vi "MQTT HASS Subscriber.vi"() -> ()   [LabVIEW 2021]
uses:
  <vilib>/LabVIEW Open Source Project/MQTT Control Packets/Control Packets/CONNECT/ConnectFlags -- cluster.ctl
  <vilib>/LabVIEW Open Source Project/MQTT Client/Client class/Client.lvclass/Client.ctl
  <vilib>/LabVIEW Open Source Project/MQTT Client/Client class/Client.lvclass
  C:/Program Files (x86)/National Instruments/LabVIEW 2021/vi.lib/LabVIEW Open Source Project/MQTT Connection/MQTT_Base/Base Class/MQTT_Base.lvclass
  <vilib>/LabVIEW Open Source Project/Connection/Connection.TCP/Connection.TCP.lvclass
  C:/Program Files (x86)/National Instruments/LabVIEW 2021/vi.lib/LabVIEW Open Source Project/Connection/Connection/Connection.lvclass
  <vilib>/LabVIEW Open Source Project/MQTT Control Packets/Control Packets/PUBLISH/PUBLISH.lvclass
  <vilib>/LabVIEW Open Source Project/MQTT Connection/MQTT_Base/Base Class/MQTT_Base.lvclass
  <vilib>/LabVIEW Open Source Project/MQTT Control Packets/Control Packets/CONNECT/CONNECT.lvclass
  <vilib>/LabVIEW Open Source Project/MQTT Control Packets/Control Packets/ControlPacket/ControlPacket.lvclass
  <vilib>/JDP Science/JDP Science Common Utilities/JDP Utility.lvlib
  <vilib>/JDP Science/JSONtext/JSONtext.lvlib
panel:
  out "Received Topic":string="homeassistant/#"
  out "Voltage Chart":dbl(graph)
  out "Current Chart":dbl(graph)
  out "State String":string
  in  "State topic":string="lab/psu/state"
  out "Config String":string
  out "Connected?":bool
  in  "Config Topic":string="homeassistant/#"
  in  "remote port (1883)":u16=1883
  in  "address (localhost)":string="localhost"
  in  "STOP":bool
  # "(Simulation)"
  # "HASS Subscriber"
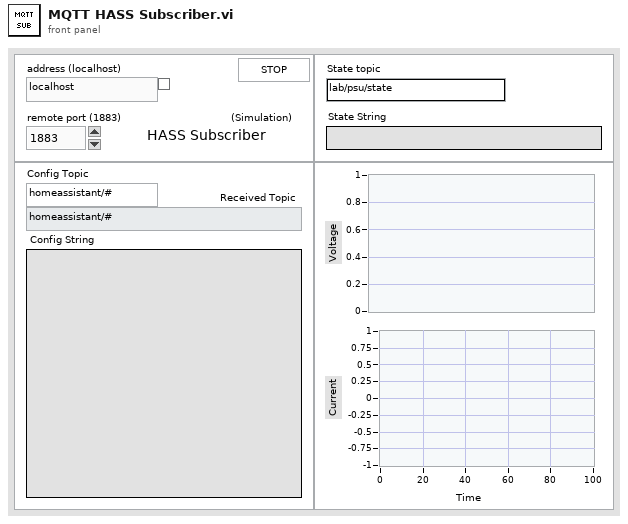
[diagram p1: front panel]
types:
  T1 = enum32{"Invalid", "Standard", "Closed", "Hidden", "Minimized", "Maximized"}
  T2 = enum32{"invalid app kind", "Development System", "Run Time System", "Student Edition", "Embedded LabVIEW", "Evaluation", "Custom"}
  T3 = cluster{"Will Topic":string, "Will Message":string, "Username":string, "Password":string}
  T4 = typedef "MQTT_Control_Packets.lvlib/CONNECT.lvclass/ConnectFlags -- cluster.ctl" = cluster{"Reserved":bool, "Clean Session":bool, "Will Flag":bool, "Will QoS 1":bool, "Will QoS 2":bool, "Will Retain":bool, "Password Flag":bool, "User Name Flag":bool}
  T5 = cluster{"Core":cluster{"Current VI Reference":refnum<vi>, "Close Panel on Exit?":bool}, "Connected?":bool}
  T6 = cluster{"Current VI Reference":refnum<vi>, "Close Panel on Exit?":bool}
  T7 = typedef "MQTT Client.lvlib/Client.lvclass/Public Events -- cluster.ctl" = cluster{"Connection Status":refnum<user-event>, "Connected":refnum<user-event>, "Application Message":refnum<user-event>}
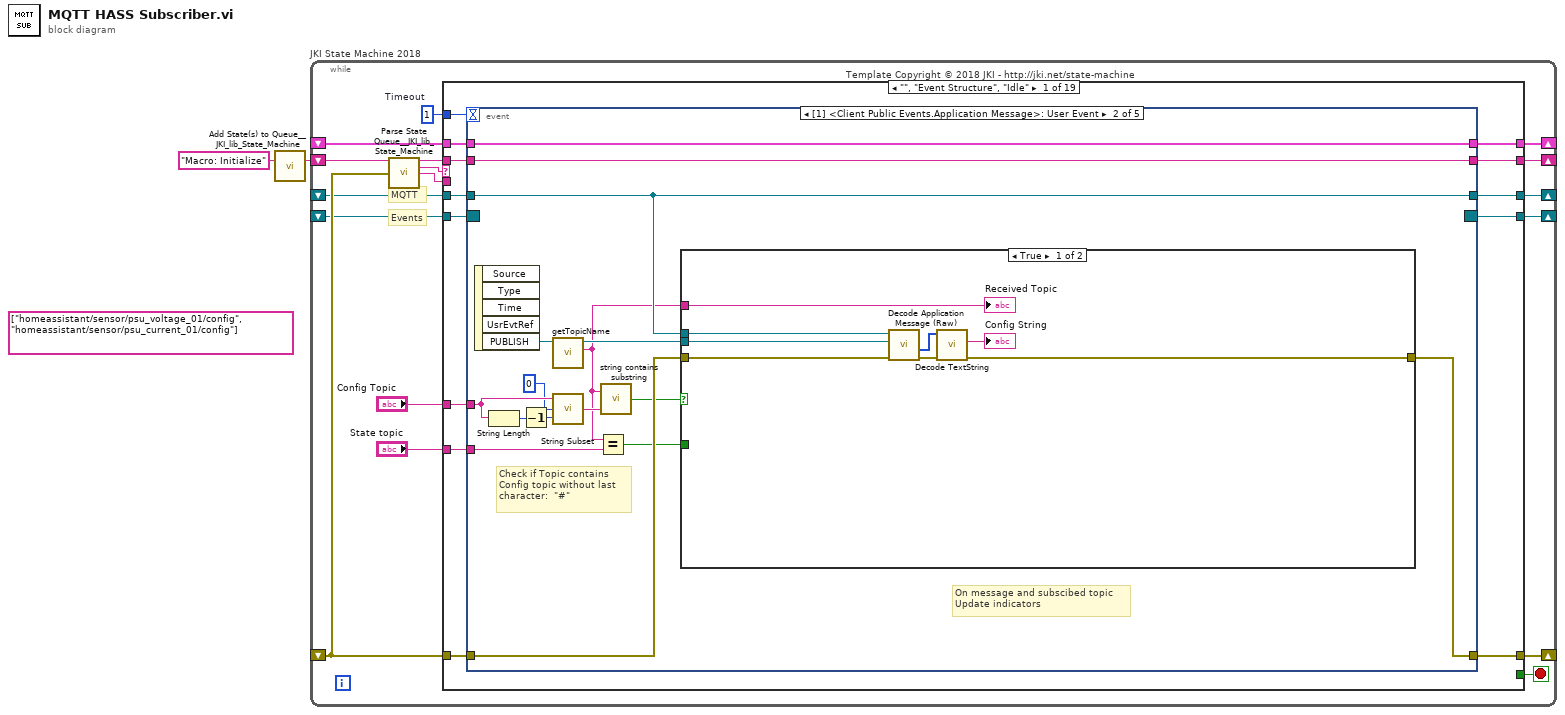
[diagram p0: block diagram]
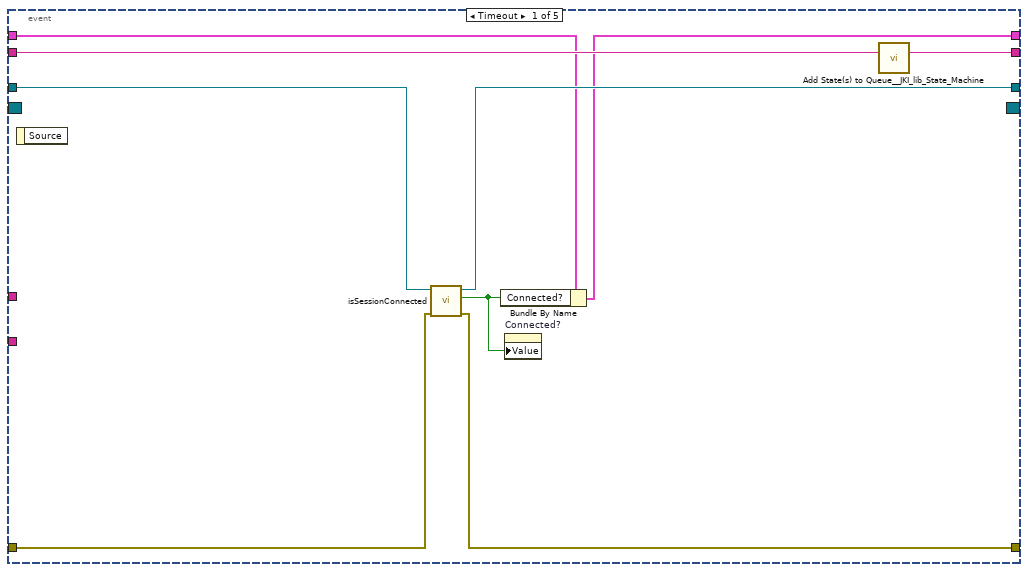
[diagram p2: hidden frame]
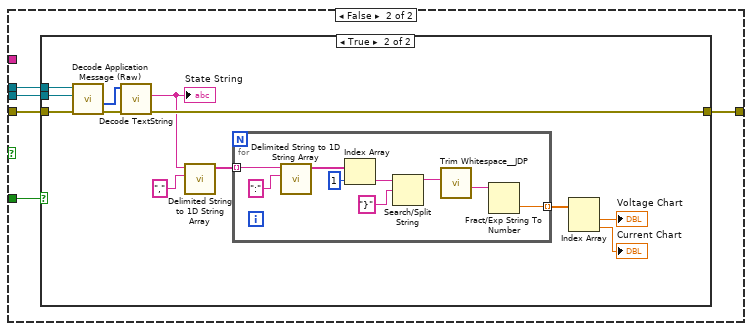
[diagram p3: hidden frame]
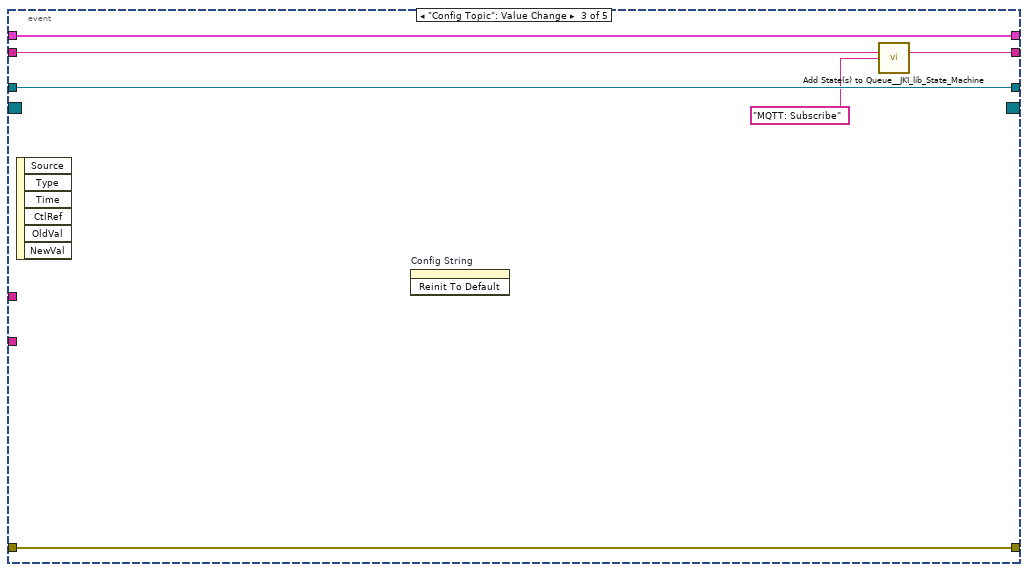
[diagram p5: hidden frame]
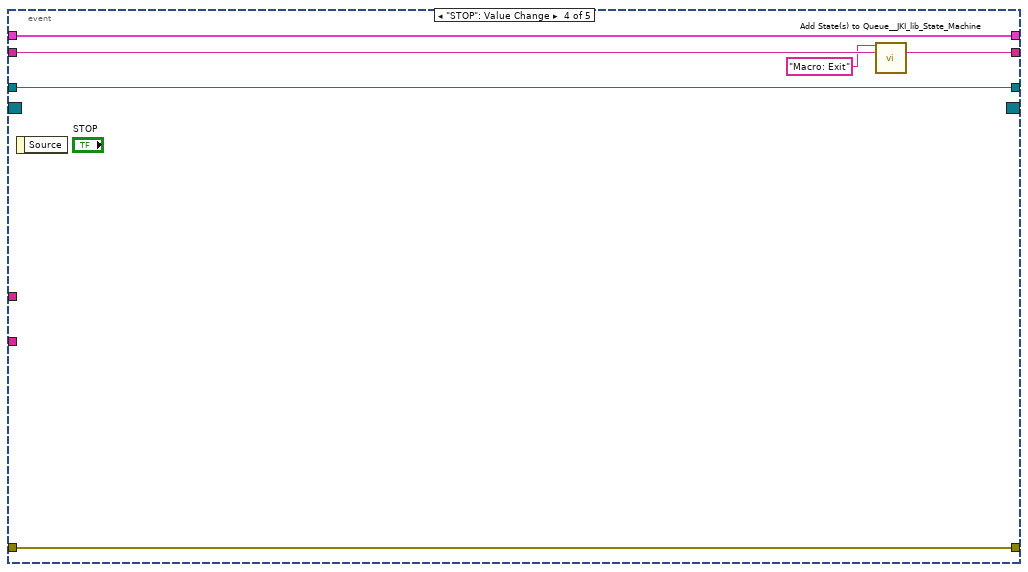
[diagram p6: hidden frame]
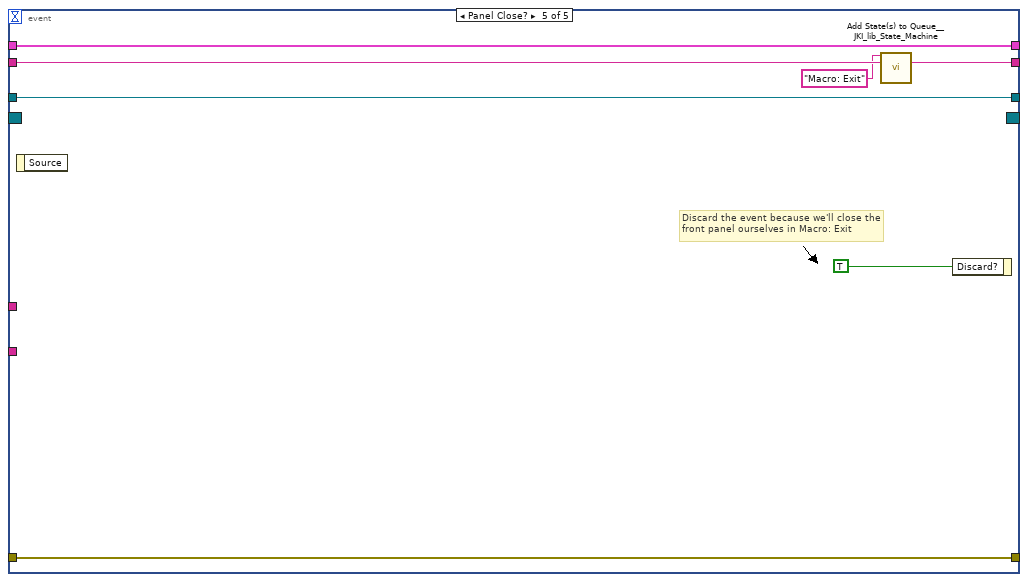
[diagram p7: hidden frame]
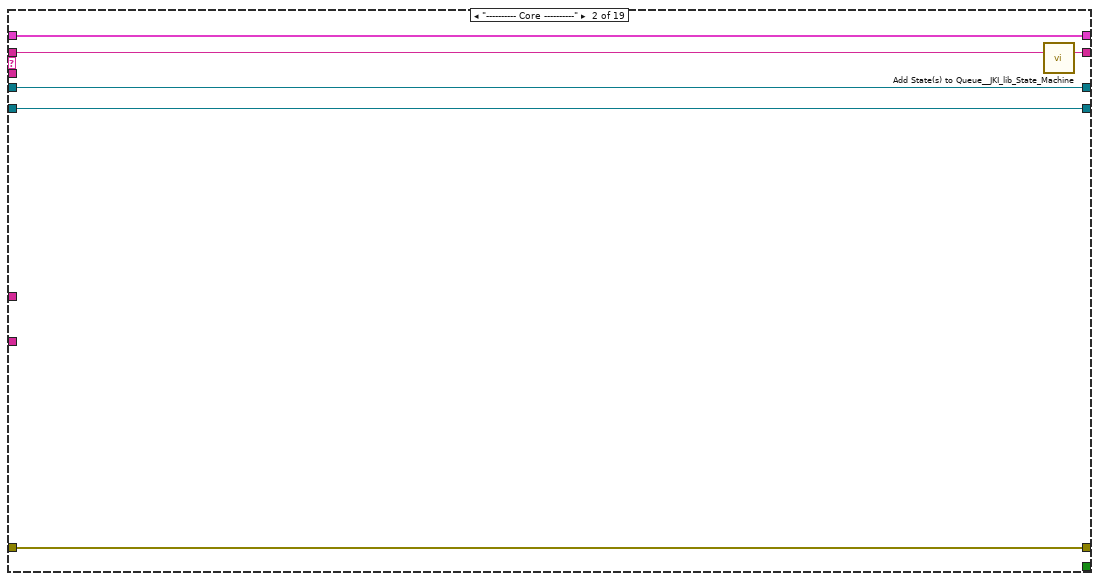
[diagram p8: hidden frame]
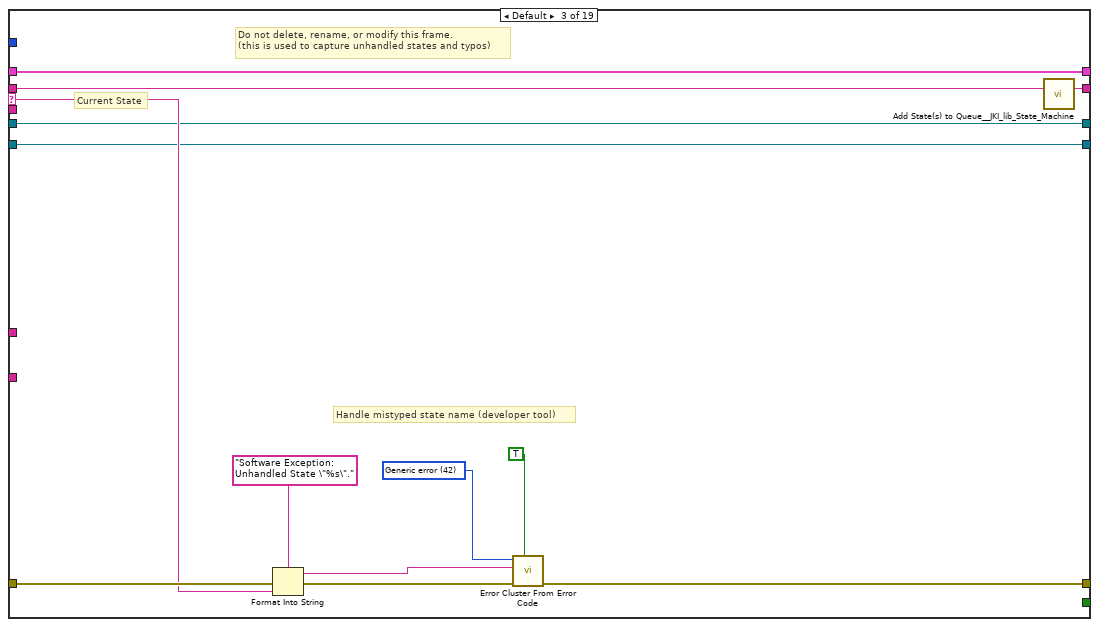
[diagram p9: hidden frame]
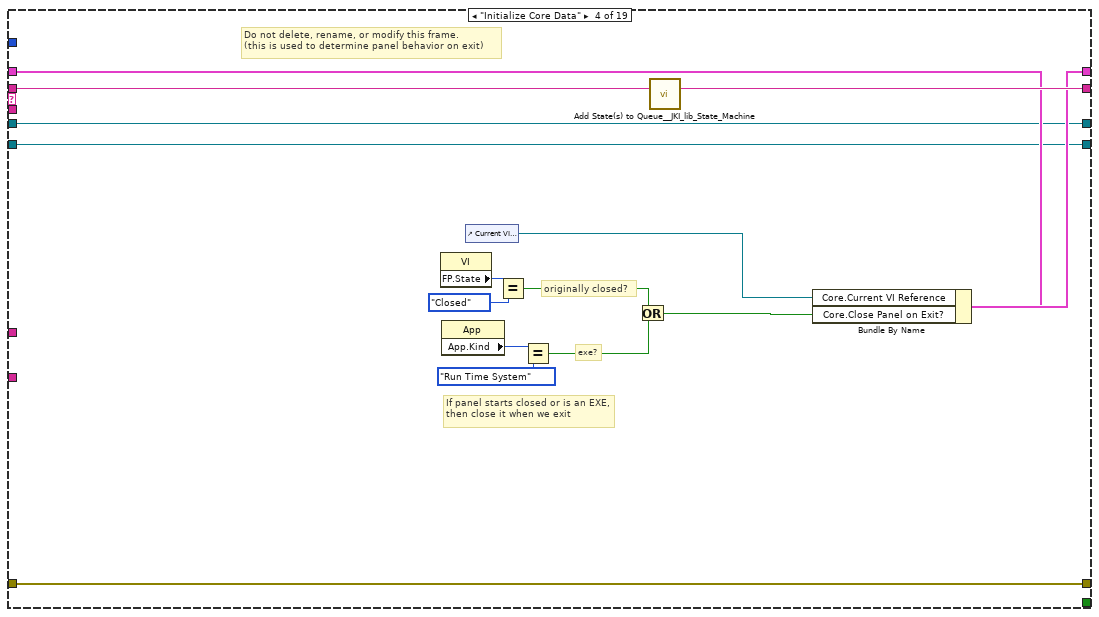
[diagram p10: hidden frame]
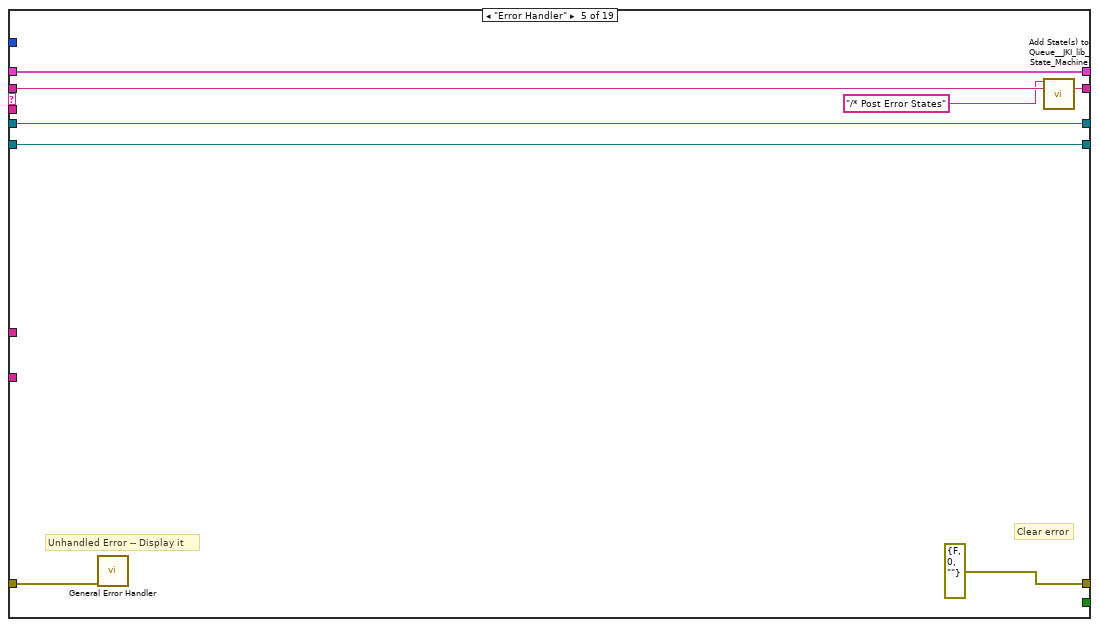
[diagram p11: hidden frame]
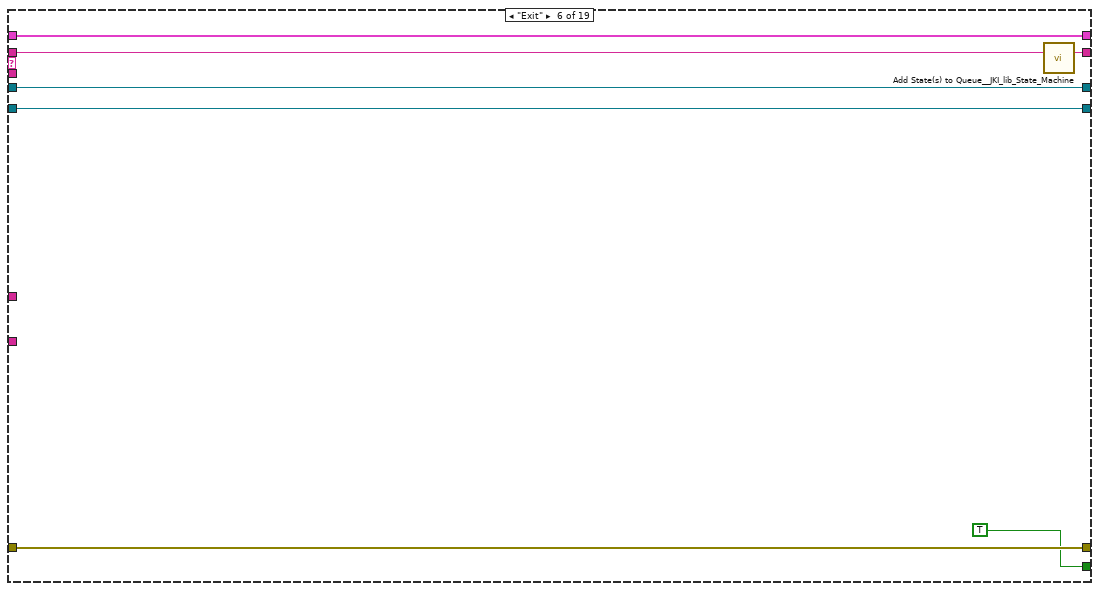
[diagram p12: hidden frame]
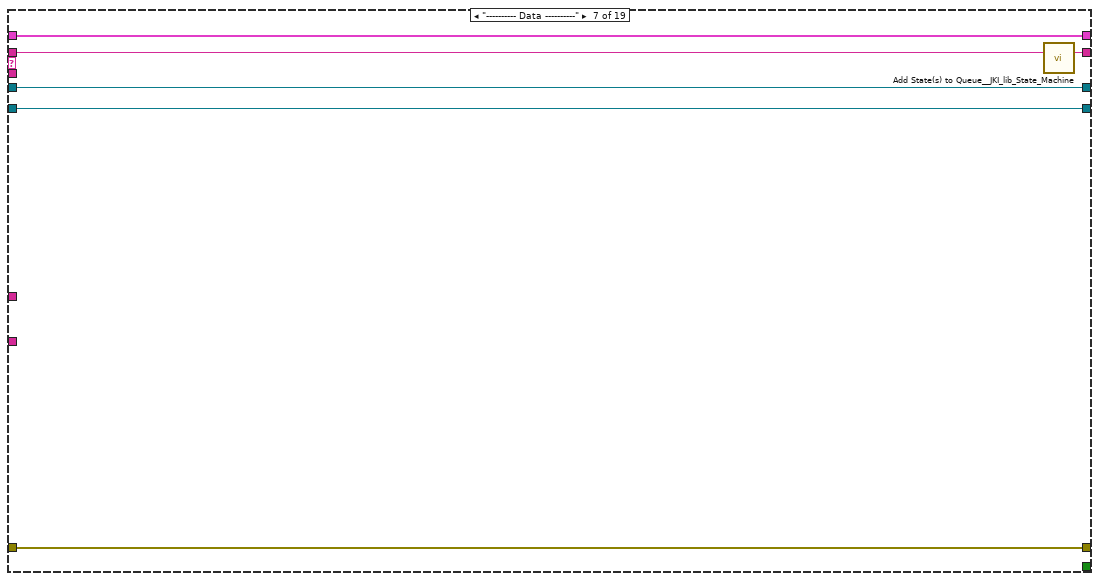
[diagram p13: hidden frame]
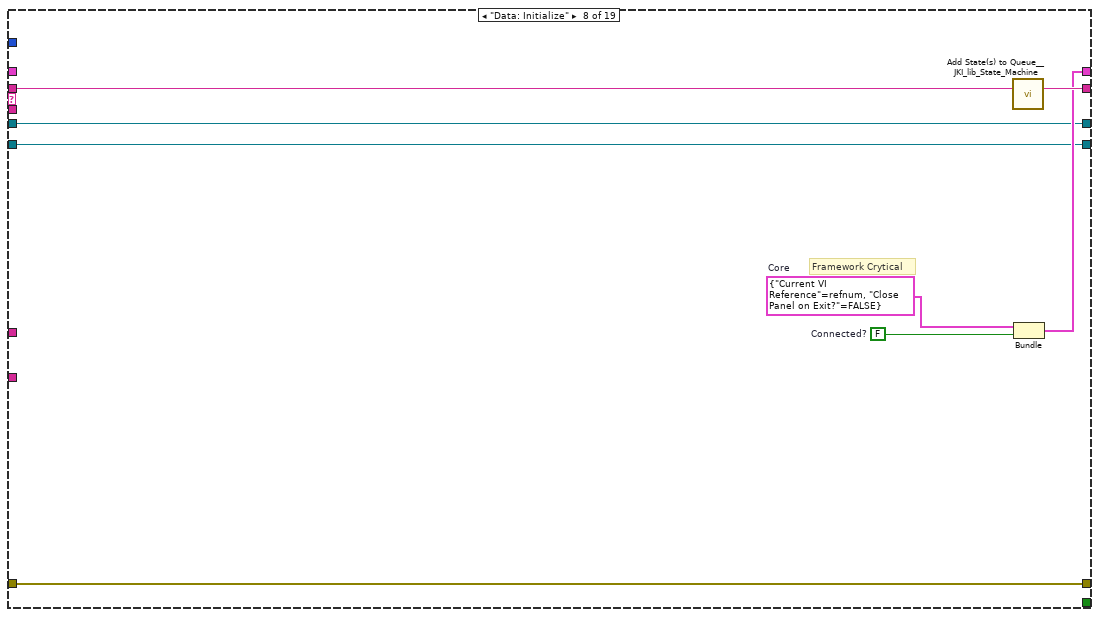
[diagram p14: hidden frame]
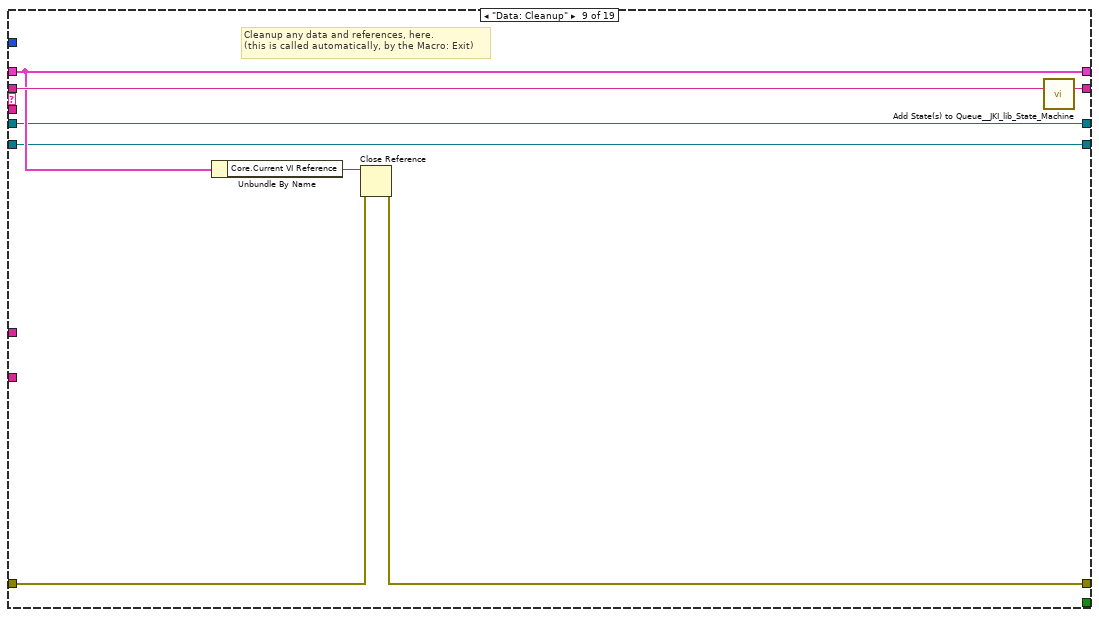
[diagram p15: hidden frame]
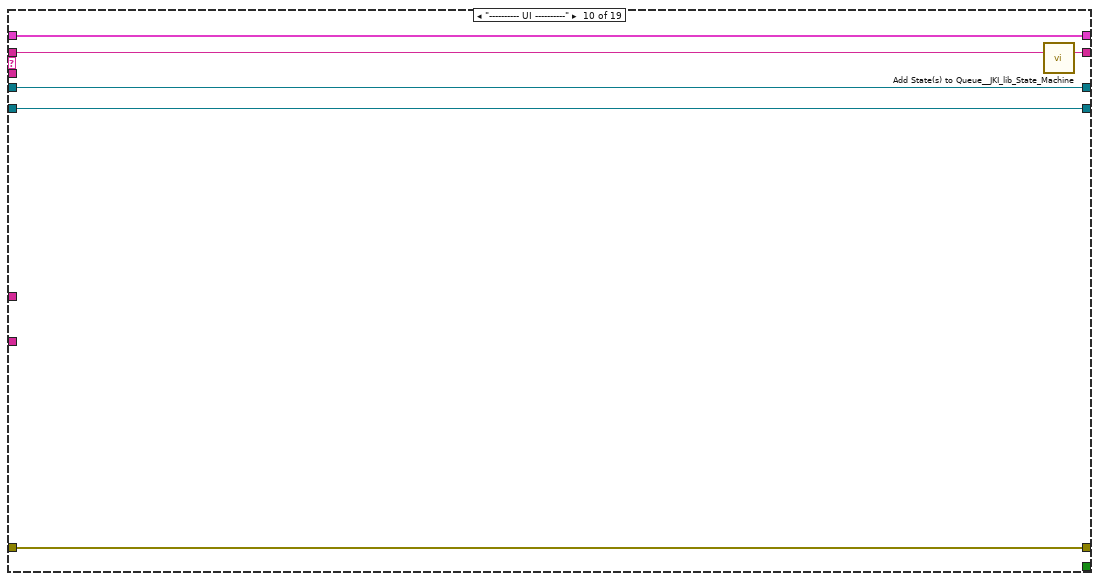
[diagram p16: hidden frame]
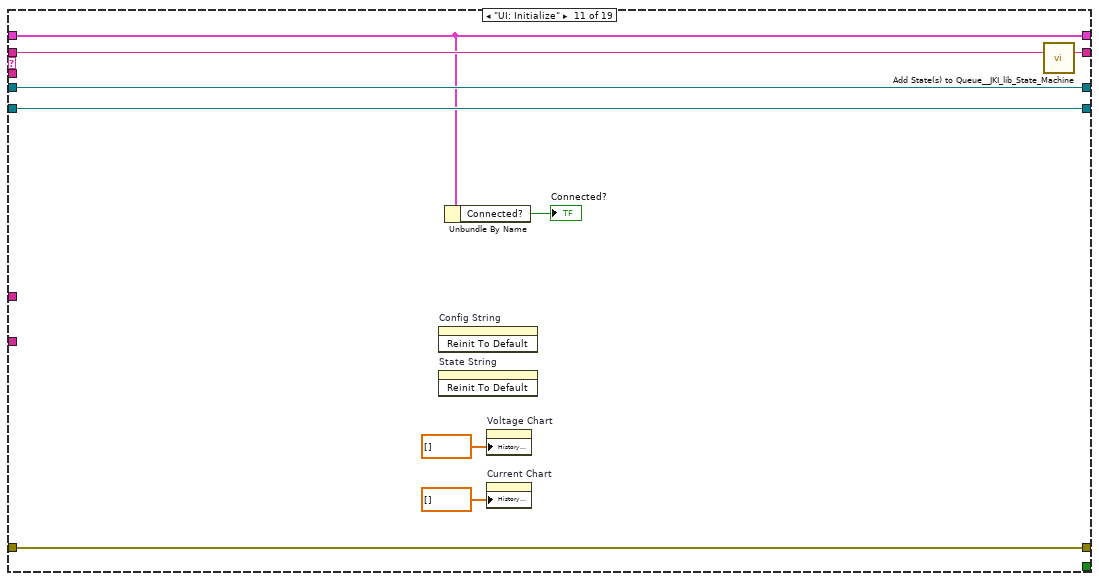
[diagram p17: hidden frame]
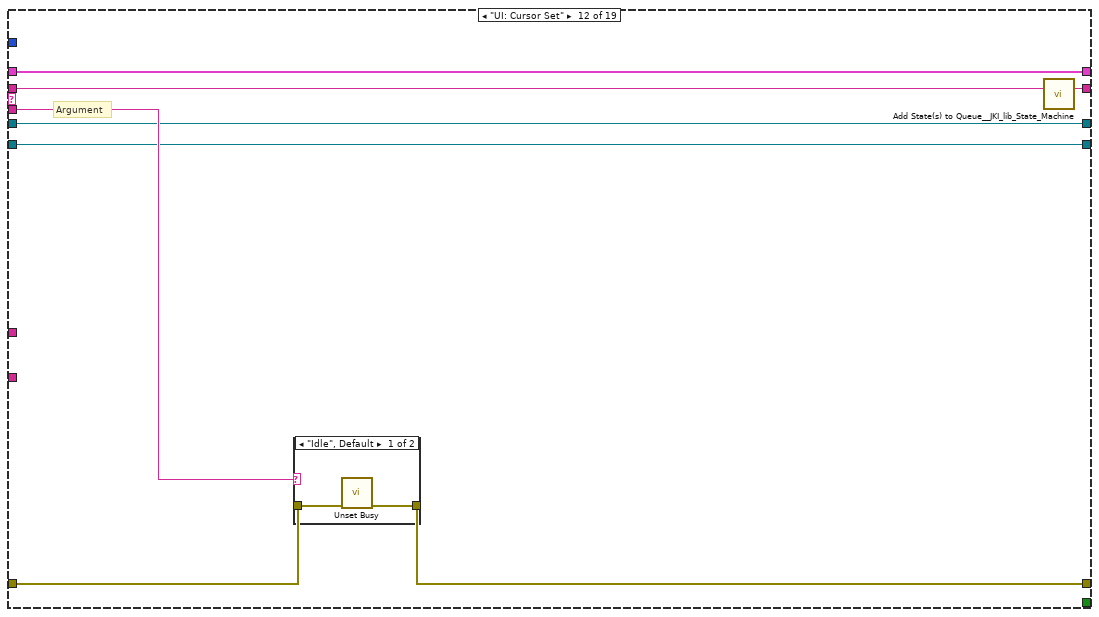
[diagram p18: hidden frame]
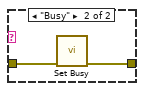
[diagram p19: hidden frame]
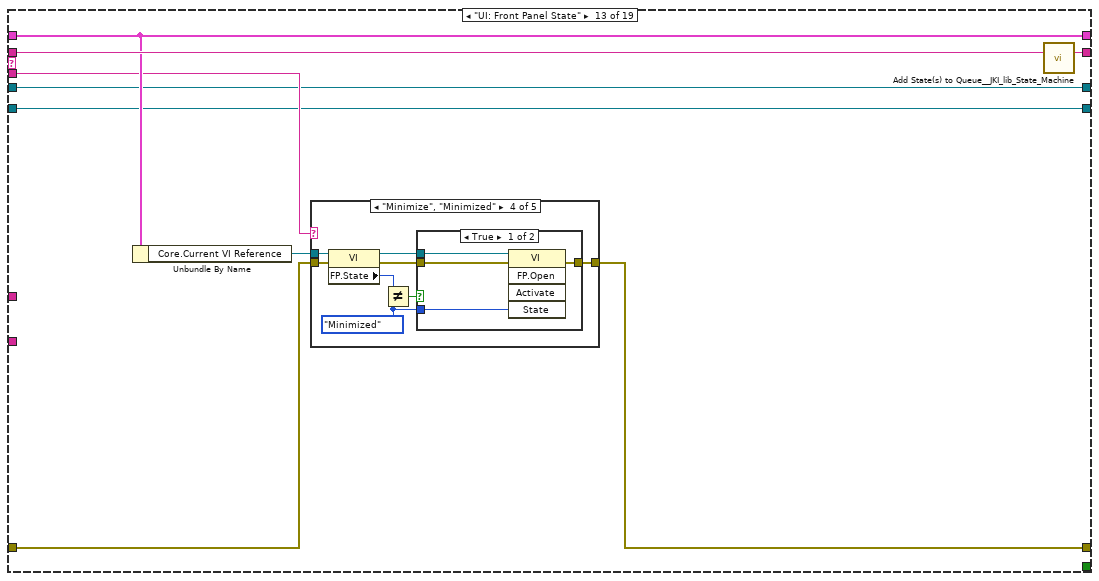
[diagram p20: hidden frame]
diagram:
  (unwired) string[] ["homeassistant/sensor/psu_voltage_01/config", "homeassistant/sensor/psu_current_01/config"]
  n1 = call <vilib>:"Add State(s) to Queue__JKI_lib_State_Machine.vi"("State(s) in (\"\")"="Macro: Initialize") -> ("States Out"=w2:string)  [unwired: 14 in]
  n2 = while "JKI State Machine 2018" {
    shift-right: [w12] -> _
    shift-left: _ -> [w11]
    shift-right: [w15] -> _
    shift-left: _ -> [w9]
    shift-right: [w14] -> _
    shift-left: w2 -> [w16]
    shift-right: [w8] -> _
    shift-left: _ -> [w7]
    shift-right: [w6] -> _
    shift-left: _ -> [w5]
    stop <- w13 stop-if-true
    w10 = 1  # Timeout
    # "Events"
    # "MQTT"
    # "Template Copyright © 2018 JKI - http://jki.net/state-machine"
    n3 = call <vilib>:"Parse State Queue__JKI_lib_State_Machine.vi"("State Queue"=w16, "Error In (no error)"=w9) -> ("Remaining States"=w18:string, "Current State"=w19:string, "Arguments"=w17:string)  [unwired: 11 in]
    n4 = case shown="\"\", \"Event Structure\", \"Idle\"" w19 {
      selector: w19 -> [_ _ w118 _ _ _ _ _ _ _ _ _ _ _ _ _ _ _ _]
      tunnel: w18 -> [w32 w115 w122 w143 w151 w158 w164 w172 w180 w186 w195 w203 w216 w287 w294 w306 w312 w340 w343]
      tunnel: w17 -> [_ _ _ _ _ _ _ _ _ _ _ w198 w210 _ _ _ _ _ _]
      tunnel: w11 -> [w30 w112 w120 w136 w148 w156 w161 _ w175 w183 w190 w201 w212 w284 w291 w303 w309 w320 w342]
      tunnel: [w29 w113 w124 w140 errorcluster {"status"=FALSE, "code"=0, "source"=""} ("error out") w155 w162 w169 w176 w184 w193 w199 w213 w285 w292 w304 w310 w322 w344] -> w15
      tunnel: w9 -> [w28 w113 w123 w140 w147 w155 w162 w169 w177 w184 w193 w200 w214 w285 w292 w304 w310 w338 w345]
      tunnel: [w31 w114 w121 w142 w150 w157 w163 w171 w179 w185 w194 w202 w215 w286 w293 w305 w311 w339 w343] -> w14
      tunnel: [_ _ _ _ _ TRUE _ _ _ _ _ _ _ _ _ _ _ _ _] -> w13
      tunnel: [w27 w112 w120 w141 w148 w156 w161 w170 w175 w183 w190 w201 w212 w284 w291 w303 w309 w319 w342] -> w12
      tunnel: w10 -> [w26 _ _ _ _ _ _ _ _ _ _ _ _ _ _ _ _ _ _]
      tunnel: [w22 w110 w116 w129 w144 w152 w159 w165 w173 w181 w191 w196 w208 w282 w288 w295 w307 w337 w352] -> w8
      tunnel: w7 -> [w23 w110 w116 w129 w144 w152 w159 w165 w173 w181 w191 w196 w208 w282 w288 w295 w307 _ w352]
      tunnel: [w24 w111 w117 w130 w145 w153 w160 w166 w174 w182 w192 w197 w209 w283 w289 w296 w308 w321 w346] -> w6
      tunnel: w5 -> [w25 w111 w117 w130 w145 w153 w160 w166 w174 w182 w192 w197 w209 w283 w289 w296 w308 _ w347]
      tunnel: "Config Topic" -> [w21 _ _ _ _ _ _ _ _ _ _ _ _ _ _ _ _ _ w348]
      tunnel: "State topic" -> [w20 _ _ _ _ _ _ _ _ _ _ _ _ _ _ _ _ _ w341]
      frame "", "Event Structure", "Idle" {
        n5 = event shown="[1] <Client Public Events.Application Message>: User Event" {
          selector: w23 -> [_ _ _ _ _]
          dyn-events: [_ _ _ _ _] -> w22
          timeout: w26 -> [_ _ _ _ _]
          tunnel: w32 -> [w41 w57 w95 w102 w109]
          tunnel: [w40 w57 w94 w101 w108] -> w31
          tunnel: w30 -> [w35 w56 w96 w99 w106]
          tunnel: [w36 w52 w93 w100 w107] -> w29
          tunnel: w28 -> [w37 w53 w93 w100 w107]
          tunnel: [w34 w56 w96 w99 w106] -> w27
          tunnel: w25 -> [w39 w54 w92 w97 w103]
          tunnel: [w38 w54 w92 w97 w103] -> w24
          tunnel: w21 -> [_ w45 _ _ _]
          tunnel: w20 -> [_ w50 _ _ _]
          event Timeout {
            n6 = event-data() -> ()  [unwired: 1 in, 1 out]
            n7 = call <vilib>:"isSessionConnected.vi"("error in (no error)"=w37, "MQTT_Base in"=w39) -> ("error out"=w36:errorcluster, "Connected?"=w33:bool, "MQTT_Base out"=w38:refnum<class "Client.lvclass">)  [unwired: 7 in]
            n8 = Bundle By Name(cluster=w35, "Connected?"=w33) -> (w34:T5)
            n9 = property on="Connected?" class="Bool (strict)"("Value"=w33) -> ()  [unwired: 2 in, 2 out]
            n10 = call <vilib>:"Add State(s) to Queue__JKI_lib_State_Machine.vi"("State(s) in (\"\")"=w41) -> ("States Out"=w40:string)  [unwired: 14 in]
          }
          event User Event {
            # "Check if Topic contains\nConfig topic without last\ncharacter:  \"#\""
            # "On message and subscibed topic\nUpdate indicators"
            n11 = event-data() -> ("PUBLISH"=w55:refnum<class "PUBLISH.lvclass">)  [unwired: 1 in, 4 out]
            n12 = String Length(string=w45) -> (length=w47:i32)
            n13 = Decrement(x=w47) -> (x-1=w44:i32)
            n14 = call <vilib>:"getTopicName.vi"("PUBLISH in"=w55) -> ("Topic"=w42:string, "PUBLISH out"=w51:refnum<class "PUBLISH.lvclass">)  [unwired: 8 in, 1 out]
            n15 = call <vilib>:"String Subset.vi"("Offset past End"=w44, "Start offset"=0, "JSON"=w45) -> ("substring"=w46:string)  [unwired: 2 in]
            n16 = Equal?(x=w42, y=w50) -> (x = y?=w49:bool)
            n17 = call "string contains substring.vi"("Search String"=w46, "Input String"=w42) -> ("Found?"=w48:bool)
            n18 = case shown="True" w48 {
              tunnel: w54 -> [w62 w67]
              tunnel: w53 -> [w64 w69]
              tunnel: [w63 w68] -> w52
              tunnel: w51 -> [w61 w66]
              tunnel: w49 -> [_ w65]
              tunnel: w42 -> [w58 _]
              frame True {
                n19 = call <vilib>:"Decode Application Message (Raw).vi"("error in (no error)"=w64, "PUBLISH"=w61, "Client in"=w62) -> ("error out"=w63:errorcluster, "Payload"=w60:u8[])  [unwired: 5 in, 2 out]
                n20 = call <vilib>:"Decode TextString.vi"("Length-Prefixed Field"=w60) -> ("Text String"=→"Config String":string)  [unwired: 8 in, 2 out]
                "Received Topic" <- w58
              }
              frame False {
                n21 = case shown="True" w65 {
                  tunnel: w69 -> [w70 w81]
                  tunnel: [w70 w80] -> w68
                  tunnel: w67 -> [_ w77]
                  tunnel: w66 -> [_ w78]
                  frame False {
                  }
                  frame True {
                    n22 = call <vilib>:"Decode Application Message (Raw).vi"("error in (no error)"=w81, "PUBLISH"=w78, "Client in"=w77) -> ("error out"=w80:errorcluster, "Payload"=w79:u8[])  [unwired: 5 in, 2 out]
                    n23 = call <vilib>:"Decode TextString.vi"("Length-Prefixed Field"=w79) -> ("Text String"=w75:string)  [unwired: 8 in, 2 out]
                    "State String" <- w75
                    n24 = call <vilib>:"Delimited String to 1D String Array.vi"("delimiter"=",", "delimited string"=w75) -> ("string array"=w74:string[])  [unwired: 9 in]
                    n25 = for {
                      tunnel: w74 -> [w83] mode=indexing
                      tunnel: [w82] -> w73 mode=indexing
                      n26 = call <vilib>:"Delimited String to 1D String Array.vi"("delimiter"=":", "delimited string"=w83) -> ("string array"=w86:string[])  [unwired: 9 in]
                      n27 = Index Array(array=w86, index=1) -> (element=w84:string)
                      n28 = Search/Split String(string=w84, search string/char (-)="}") -> (substring before match=w89:string)  [unwired: 1 in, 2 out]
                      n29 = call <vilib>:"Trim Whitespace__JDP.vi"("String in"=w89) -> ("String out"=w88:string)  [unwired: 6 in]
                      n30 = Fract/Exp String To Number(string=w88) -> (number=w82:dbl)  [unwired: 3 in, 1 out]
                    }
                    n31 = Index Array(array=w73) -> (element #1=→"Voltage Chart":dbl, element #2=→"Current Chart":dbl)  [unwired: 2 in]
                  }
                }
              }
            }
          }
          event "Config Topic": Value Change {
            n32 = event-data() -> ()  [unwired: 1 in, 6 out]
            n33 = invoke on="Config String" class="Str" method="Reinit To Default"() -> ()  [unwired: 3 in, 3 out]
            n34 = call <vilib>:"Add State(s) to Queue__JKI_lib_State_Machine.vi"("State(s) in (\"\")"=w95, "State(s) at Back (\"\")"="MQTT: Subscribe" ("State(s) at Back (\"\")")) -> ("States Out"=w94:string)  [unwired: 13 in]
          }
          event "STOP": Value Change {
            n35 = event-data() -> ()  [unwired: 1 in, 1 out]
            n36 = call <vilib>:"Add State(s) to Queue__JKI_lib_State_Machine.vi"("State(s) in Front (\"\")"="Macro: Exit", "State(s) in (\"\")"=w102) -> ("States Out"=w101:string)  [unwired: 13 in]
          }
          event Panel Close? {
            # "Discard the event because we'll close the front panel ourselves in Macro: Exit"
            n37 = event-data() -> ()  [unwired: 1 in, 1 out]
            n38 = call <vilib>:"Add State(s) to Queue__JKI_lib_State_Machine.vi"("State(s) in Front (\"\")"="Macro: Exit", "State(s) in (\"\")"=w109) -> ("States Out"=w108:string)  [unwired: 13 in]
            n39 = event-data("Discard?"=TRUE) -> ()  [unwired: 1 in, 1 out]
          }
        }
      }
      frame "---------- Core ----------" {
        n40 = call <vilib>:"Add State(s) to Queue__JKI_lib_State_Machine.vi"("State(s) in (\"\")"=w115) -> ("States Out"=w114:string)  [unwired: 14 in]
      }
      frame Default {
        w127 = 42 items=["No error", "Argument error", "Memory is full", "Out of zone", "End of file", "File already open", "Generic file I/O error", "File not found", "File permission error", "Disk is full", "Duplicate path", "Too many files open", "System feature not enabled", "Resource file not found", "Cannot add resource", "Resource not found", "Image not found", "Image memory error", "Pen does not exist", "Config type invalid", "Config token not found", "Config parse error", "Config memory error", "Bad external code format", "Bad external code offset", "External code not present", "Null window", "Destroy window error", "Null menu", "Print aborted", "Bad print record", "Print driver error", "Windows error during printing", "Memory error during printing", "Print dialog error", "Generic print error", "Invalid device refnum", "Device not found", "Device parameter error", "Device unit error", "Cannot open device", "Device call aborted", "Generic error", "Cancelled by user", "Object ID too low", "Object ID too high", "Object not in heap", "Unknown heap", "Unknown object (invalid DefProc)", "Unknown object (DefProc not in table)", "Message out of range", "Invalid (null) method", "Unknown message", "Manager call not supported", "Bad address", "Network operation in progress", "Network operation timed out", "Connection is busy", "Network attribute not supported", "Network error", "Address in use", "System out of memory", "Connection aborted", "Connection refused", "Not connected", "Already connected", "Connection closed", "Initialization error (interapplication manager)", "Bad occurrence", "Wait on unbound occurrence handler", "Occurrence queue overflow", "Datalog type conflict", "Unused", "Unrecognized type (interapplication manager)", "Memory corrupt", "Failed to make temporary DLL", "Old CIN version", "Drag socket not found", "Failed to load drop-object", "Failed to register OLE object", "Failed to release OLE object", "Format specifier type mismatch", "Unknown format specifier", "Too few format specifiers", "Too many format specifiers", "Scan failed", "Newer CIN version", "Error converting to variant", "Runtime menu error", "Password tampered", "Variant attribute not found", "Incompatible variant data type", "Event data is not available", "Event Store is not present", "Occurrence is not found", "Event Queue is not created", "Event info is not available", "Refnum passed is NULL", "Error retrieving Class GUID", "Error retrieving CoClass GUID", "Error retrieving TypeLib GUID.", "Bad built application magic bytes.", "Specific driver is different from the specific driver associated with the Logical Name.", "There is no session opened to the class driver.", "Max Error", "MAX - Error with config objects", "MAX - Error loading configuration", "MAX - Group not supported"]
        # "Current State"
        # "Do not delete, rename, or modify this frame.\n(this is used to capture unhandled states and typos)"
        # "Handle mistyped state name (developer tool)"
        n41 = Format Into String(format string="Software Exception: Unhandled State \"%s\"." ("message"), error in=w123, w118) -> (resulting string=w126:string, error out=w125:errorcluster)  [unwired: 1 in]
        n42 = call <vilib>:"Error Cluster From Error Code.vi"("show call chain? (False)"=TRUE, "error in (no error)"=w125, "error message (\"\")"=w126, "error code (0)"=w127) -> ("error out"=w124:errorcluster)  [unwired: 5 in]
        n43 = call <vilib>:"Add State(s) to Queue__JKI_lib_State_Machine.vi"("State(s) in (\"\")"=w122) -> ("States Out"=w121:string)  [unwired: 14 in]
      }
      frame "Initialize Core Data" {
        # "Do not delete, rename, or modify this frame.\n(this is used to determine panel behavior on exit)"
        # "originally closed?"
        # "exe?"
        # "If panel starts closed or is an EXE, then close it when we exit"
        n44 = property class="VI"() -> ("FP.State"=w133:T1)  [unwired: 2 in, 2 out]
        n45 = property class="App"() -> ("App.Kind"=w139:T2)  [unwired: 2 in, 2 out]
        n46 = control-ref of="Current VI Reference"() -> (w134:refnum<vi>)
        n47 = Equal?(x=w133, y=T1."Closed" ("Front Panel Window:State")) -> (x = y?=w131:bool)
        n48 = Equal?(x=w139, y=T2."Run Time System" ("Application:Kind")) -> (x = y?=w137:bool)
        n49 = Or(x=w131, y=w137) -> (x .or. y?=w135:bool)
        n50 = call <vilib>:"Add State(s) to Queue__JKI_lib_State_Machine.vi"("State(s) in (\"\")"=w143) -> ("States Out"=w142:string)  [unwired: 14 in]
        n51 = Bundle By Name(cluster=w136, "Core.Current VI Reference"=w134, "Core.Close Panel on Exit?"=w135) -> (w141:T5)
      }
      frame "Error Handler" {
        # "Unhandled Error -- Display it"
        # "Clear error"
        n52 = call <vilib>:"General Error Handler.vi"("error in (no error)"=w147) -> ()  [unwired: 10 in, 5 out]
        n53 = call <vilib>:"Add State(s) to Queue__JKI_lib_State_Machine.vi"("State(s) in Front (\"\")"="/* Post Error States", "State(s) in (\"\")"=w151) -> ("States Out"=w150:string)  [unwired: 13 in]
      }
      frame "Exit" {
        n54 = call <vilib>:"Add State(s) to Queue__JKI_lib_State_Machine.vi"("State(s) in (\"\")"=w158) -> ("States Out"=w157:string)  [unwired: 14 in]
      }
      frame "---------- Data ----------" {
        n55 = call <vilib>:"Add State(s) to Queue__JKI_lib_State_Machine.vi"("State(s) in (\"\")"=w164) -> ("States Out"=w163:string)  [unwired: 14 in]
      }
      frame "Data: Initialize" {
        w167 = T6 {"Current VI Reference"=refnum, "Close Panel on Exit?"=FALSE}  # Core
        w168 = FALSE  # Connected?
        # "Framework Crytical"
        n56 = call <vilib>:"Add State(s) to Queue__JKI_lib_State_Machine.vi"("State(s) in (\"\")"=w172) -> ("States Out"=w171:string)  [unwired: 14 in]
        n57 = Bundle("Core"=w167, "Connected?"=w168) -> (w170:T5)  [unwired: 1 in]
      }
      frame "Data: Cleanup" {
        # "Cleanup any data and references, here.\n(this is called automatically, by the Macro: Exit)"
        n58 = Unbundle By Name(w175) -> ("Core.Current VI Reference"=w178:refnum<vi>)
        n59 = Close Reference(reference=w178, error in (no error)=w177) -> (error out=w176:errorcluster)
        n60 = call <vilib>:"Add State(s) to Queue__JKI_lib_State_Machine.vi"("State(s) in (\"\")"=w180) -> ("States Out"=w179:string)  [unwired: 14 in]
      }
      frame "---------- UI ----------" {
        n61 = call <vilib>:"Add State(s) to Queue__JKI_lib_State_Machine.vi"("State(s) in (\"\")"=w186) -> ("States Out"=w185:string)  [unwired: 14 in]
      }
      frame "UI: Initialize" {
        n62 = invoke on="Config String" class="Str" method="Reinit To Default"() -> ()  [unwired: 3 in, 3 out]
        n63 = invoke on="State String" class="Str" method="Reinit To Default"() -> ()  [unwired: 3 in, 3 out]
        n64 = Unbundle By Name(w190) -> ("Connected?"=→"Connected?":bool)
        n65 = property on="Voltage Chart" class="WFChart (strict)"("History Data"=dbl[] []) -> ()  [unwired: 2 in, 2 out]
        n66 = property on="Current Chart" class="WFChart (strict)"("History Data"=dbl[] []) -> ()  [unwired: 2 in, 2 out]
        n67 = call <vilib>:"Add State(s) to Queue__JKI_lib_State_Machine.vi"("State(s) in (\"\")"=w195) -> ("States Out"=w194:string)  [unwired: 14 in]
      }
      frame "UI: Cursor Set" {
        # "Argument"
        n68 = case shown="\"Idle\", Default" w198 {
          tunnel: w200 -> [w205 w207]
          tunnel: [w204 w206] -> w199
          frame "Idle", Default {
            n69 = call <vilib>:"Unset Busy.vi"("error in (no error)"=w205) -> ("error out"=w204:errorcluster)  [unwired: 10 in]
          }
          frame "Busy" {
            n70 = call <vilib>:"Set Busy.vi"("error in (no error)"=w207) -> ("error out"=w206:errorcluster)  [unwired: 9 in, 1 out]
          }
        }
        n71 = call <vilib>:"Add State(s) to Queue__JKI_lib_State_Machine.vi"("State(s) in (\"\")"=w203) -> ("States Out"=w202:string)  [unwired: 14 in]
      }
      frame "UI: Front Panel State" {
        n72 = Unbundle By Name(w212) -> ("Core.Current VI Reference"=w211:refnum<vi>)
        n73 = case shown="\"Minimize\", \"Minimized\"" w210 {
          tunnel: w214 -> [w222 w237 w248 w261 w274]
          tunnel: [w224 w238 w250 w263 w276] -> w213
          tunnel: w211 -> [w223 w235 w249 w262 w275]
          frame "Open", "Standard", Default {
            w217 = T1."Standard" ("State")
            n74 = property class="VI"(reference=w223, error in=w222) -> (reference out=w220:refnum<vi>, error out=w221:errorcluster, "FP.State"=w219:T1)
            n75 = Not Equal?(x=w219, y=w217) -> (x != y?=w218:bool)
            n76 = case shown="True" w218 {
              tunnel: [w228 w230] -> w224
              tunnel: w221 -> [w227 w230]
              tunnel: w220 -> [w226 _]
              tunnel: w217 -> [w225 _]
              frame True {
                n77 = invoke class="VI" method="FP.Open"(reference=w226, error in=w227, "Activate"=TRUE, "State"=w225) -> (error out=w228:errorcluster)  [unwired: 1 in, 4 out]
              }
              frame False {
              }
            }
          }
          frame "Close", "Closed" {
            n78 = property class="VI"(reference=w235, error in=w237) -> (reference out=w234:refnum<vi>, error out=w236:errorcluster, "FP.State"=w232:T1)
            n79 = Not Equal?(x=w232, y=T1."Closed" ("Front Panel Window:State")) -> (x != y?=w231:bool)
            n80 = case shown="True" w231 {
              tunnel: [w239 w242] -> w238
              tunnel: w236 -> [w239 w241]
              tunnel: w234 -> [_ w240]
              frame False {
              }
              frame True {
                n81 = invoke class="VI" method="FP.Close"(reference=w240, error in=w241) -> (error out=w242:errorcluster)  [unwired: 1 in, 2 out]
              }
            }
          }
          frame "Hidden", "Hide" {
            w243 = T1."Hidden" ("State")
            n82 = property class="VI"(reference=w249, error in=w248) -> (reference out=w246:refnum<vi>, error out=w247:errorcluster, "FP.State"=w245:T1)
            n83 = Not Equal?(x=w245, y=w243) -> (x != y?=w244:bool)
            n84 = case shown="True" w244 {
              tunnel: [w254 w255] -> w250
              tunnel: w247 -> [w253 w255]
              tunnel: w246 -> [w252 _]
              tunnel: w243 -> [w251 _]
              frame True {
                n85 = invoke class="VI" method="FP.Open"(reference=w252, error in=w253, "State"=w251) -> (error out=w254:errorcluster)  [unwired: 2 in, 4 out]
              }
              frame False {
              }
            }
          }
          frame "Minimize", "Minimized" {
            w256 = T1."Minimized" ("State")
            n86 = property class="VI"(reference=w262, error in=w261) -> (reference out=w259:refnum<vi>, error out=w260:errorcluster, "FP.State"=w258:T1)
            n87 = Not Equal?(x=w258, y=w256) -> (x != y?=w257:bool)
            n88 = case shown="True" w257 {
              tunnel: [w267 w268] -> w263
              tunnel: w260 -> [w266 w268]
              tunnel: w259 -> [w265 _]
              tunnel: w256 -> [w264 _]
              frame True {
                n89 = invoke class="VI" method="FP.Open"(reference=w265, error in=w266, "State"=w264) -> (error out=w267:errorcluster)  [unwired: 2 in, 4 out]
              }
              frame False {
              }
            }
          }
          frame "Maximize", "Maximized" {
            w269 = T1."Maximized" ("State")
            n90 = property class="VI"(reference=w275, error in=w274) -> (reference out=w272:refnum<vi>, error out=w273:errorcluster, "FP.State"=w271:T1)
            n91 = Not Equal?(x=w271, y=w269) -> (x != y?=w270:bool)
            n92 = case shown="True" w270 {
              tunnel: [w280 w281] -> w276
              tunnel: w273 -> [w279 w281]
              tunnel: w272 -> [w278 _]
              tunnel: w269 -> [w277 _]
              frame True {
                n93 = invoke class="VI" method="FP.Open"(reference=w278, error in=w279, "State"=w277) -> (error out=w280:errorcluster)  [unwired: 2 in, 4 out]
              }
              frame False {
              }
            }
          }
        }
        n94 = call <vilib>:"Add State(s) to Queue__JKI_lib_State_Machine.vi"("State(s) in (\"\")"=w216) -> ("States Out"=w215:string)  [unwired: 14 in]
      }
      frame "---------- Macro ----------" {
        n95 = call <vilib>:"Add State(s) to Queue__JKI_lib_State_Machine.vi"("State(s) in (\"\")"=w287) -> ("States Out"=w286:string)  [unwired: 14 in]
      }
      frame "Macro: Initialize" {
        n96 = call <vilib>:"Add State(s) to Queue__JKI_lib_State_Machine.vi"("State(s) in Front (\"\")"="Data: Initialize\nInitialize Core Data\nMQTT: Initialize\nUI: Initialize\nUI: Front Panel State >> Open", "State(s) in (\"\")"=w294) -> ("States Out"=w293:string)  [unwired: 13 in]
      }
      frame "Macro: Exit" {
        n97 = Unbundle By Name(w303) -> ("Core.Close Panel on Exit?"=w302:bool)
        n98 = Select(t="UI: Front Panel State >> Close", s=w302, f="") -> (s? t:f=w299:string)
        n99 = call <vilib>:"Add State(s) to Queue__JKI_lib_State_Machine.vi"("State(s) in (\"\")"=w299, "State(s) at Back (\"\")"="Data: Cleanup\nExit") -> ("States Out"=w297:string)  [unwired: 13 in]
        n100 = call <vilib>:"Add State(s) to Queue__JKI_lib_State_Machine.vi"("State(s) in Front (\"\")"=w297, "State(s) in (\"\")"=w306) -> ("States Out"=w305:string)  [unwired: 13 in]
      }
      frame "---------- MQTT Broker ----------" {
        n101 = call <vilib>:"Add State(s) to Queue__JKI_lib_State_Machine.vi"("State(s) in (\"\")"=w312) -> ("States Out"=w311:string)  [unwired: 14 in]
      }
      frame "MQTT: initialize" {
        # "Exit on fail"
        # "Connect"
        n102 = call <vilib>:"Configure TCP Connection.vi"("error in (no error)"=w338, "remote port (80)"="remote port (1883)", "address (localhost)"="address (localhost)") -> ("error out"=w333:errorcluster, "Connection.TCP"=w332:refnum<class "Connection.TCP.lvclass">)  [unwired: 7 in]
        n103 = call <vilib>:"Create MQTT Client.vi"("error in (no error)"=w333, "Connection Configuration"=w332) -> ("error out"=w330:errorcluster, "Client out"=w331:refnum<class "Client.lvclass">)  [unwired: 8 in]
        n104 = call <vilib>:"Read Public Events.vi"("error in (no error)"=w330, "Client in"=w331) -> ("error out"=w328:errorcluster, "Client Public Events"=w329:T7, "Client out"=w327:refnum<class "Client.lvclass">)  [unwired: 7 in]
        n105 = register-events(error in=w328, w329) -> (reference out=w337:refnum<event-registration>, error out=w336:errorcluster)  [unwired: 1 in]
        n106 = call <vilib>:"Start.vi"("error in (no error)"=w336, "MQTT_Base in"=w327) -> ("error out"=w325:errorcluster, "MQTT_Base out"=w326:refnum<class "Client.lvclass">)  [unwired: 7 in, 1 out]
        n107 = call <vilib>:"Connect to Server.vi"("Connect Flags"=T4 {"Reserved"=FALSE, "Clean Session"=TRUE, "Will Flag"=FALSE, "Will QoS 1"=FALSE, "Will QoS 2"=FALSE, "Will Retain"=FALSE, "Password Flag"=TRUE, "User Name Flag"=TRUE}, "Payload"=T3 {"Will Topic"="", "Will Message"="", "Username"="username", "Password"="password"}, "error in (no error)"=w325, "Client in"=w326) -> ("error out"=w323:errorcluster, "Client out"=w324:refnum<class "Client.lvclass">)  [unwired: 4 in, 2 out]
        n108 = call <vilib>:"isSessionConnected.vi"("error in (no error)"=w323, "MQTT_Base in"=w324) -> ("error out"=w322:errorcluster, "Connected?"=w316:bool, "MQTT_Base out"=w321:refnum<class "Client.lvclass">)  [unwired: 7 in]
        n109 = Select(t="MQTT: Subscribe", s=w316, f="Macro: Exit" ("State(s) at Back (\"\")")) -> (s? t:f=w315:string)
        n110 = Bundle By Name(cluster=w320, "Connected?"=w316) -> (w319:T5)
        n111 = call <vilib>:"Add State(s) to Queue__JKI_lib_State_Machine.vi"("State(s) in (\"\")"=w340, "State(s) at Back (\"\")"=w315) -> ("States Out"=w339:string)  [unwired: 13 in]
      }
      frame "MQTT: Subscribe" {
        n112 = call <vilib>:"isSessionConnected.vi"("error in (no error)"=w345, "MQTT_Base in"=w347) -> ("error out"=w350:errorcluster, "Connected?"=w349:bool, "MQTT_Base out"=w351:refnum<class "Client.lvclass">)  [unwired: 7 in]
        n113 = property on="Connected?" class="Bool (strict)"("Value"=w349) -> ()  [unwired: 2 in, 2 out]
        n114 = case shown="True" w349 {
          tunnel: w351 -> [w354 w362]
          tunnel: w350 -> [w353 w361]
          tunnel: [w353 w357] -> w344
          tunnel: [w354 w356] -> w346
          tunnel: w348 -> [_ w360]
          tunnel: w341 -> [_ w355]
          frame False {
          }
          frame True {
            # "Config"
            # "State"
            n115 = call <vilib>:"Subscribe (Scalar).vi"("error in (no error)"=w361, "Topic Filter"=w360, "Client in"=w362) -> ("error out"=w358:errorcluster, "Client out"=w359:refnum<class "Client.lvclass">)  [unwired: 6 in, 1 out]
            n116 = call <vilib>:"Subscribe (Scalar).vi"("error in (no error)"=w358, "Topic Filter"=w355, "Client in"=w359) -> ("error out"=w357:errorcluster, "Client out"=w356:refnum<class "Client.lvclass">)  [unwired: 6 in, 1 out]
          }
        }
      }
    }
  }
